vi "Pressure Read Single.vi"(8 "error in":errorcluster, 9 "Channel Index":i32=1, 11 "Chiller in":refnum<class "Chiller.lvclass">) -> (0 "error out":errorcluster, 1 "Changed or First Call?":bool, 2 "Pressure SP":dbl, 3 "Chiller out":refnum<class "Chiller.lvclass">)   [LabVIEW 2023, in "Chiller.lvclass"]
uses:
  Chiller.lvclass
  Low Level Capabilities/Pressure/Pressure Setpoint/Pressure Setpoint.lvclass
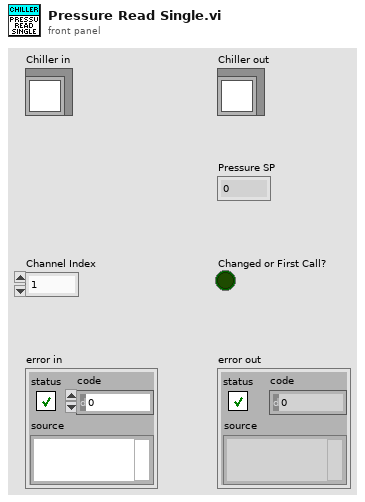
[diagram p1: front panel]
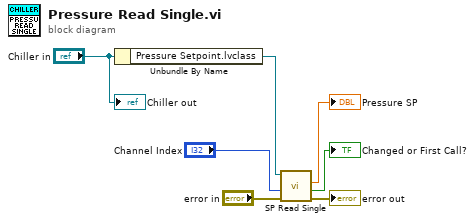
[diagram p0: block diagram]
diagram:
  n1 = Unbundle By Name("Chiller in") -> ("Pressure Setpoint.lvclass"=w7:refnum<class "Pressure Setpoint.lvclass">)
  n2 = call-dynamic "SP Read Single.vi"("error in"="error in", "Channel Index"="Channel Index", "Pressure Setpoint in"=w7) -> ("error out"=→"error out":errorcluster, "Changed or First Call?"=→"Changed or First Call?":bool, "Pressure SP"=→"Pressure SP":dbl)  [unwired: 5 in, 1 out]
  "Chiller out" <- "Chiller in"
